vi "LH_DeleteIndexedContent.vi"(0 "InputList":refnum<class "ListHead.lvclass">, 1 "Index":i32) -> (2 "OutputList":refnum<class "ListHead.lvclass">, 3 "OutputContent":i32, 4 "IsEmpty?":bool)   [LabVIEW 2014, in "ListHead.lvclass"]
uses:
  ListHead.lvclass
  ListHead.lvclass/ListHead.ctl
  ListNode.lvclass
  ListNodeVirtual.lvclass
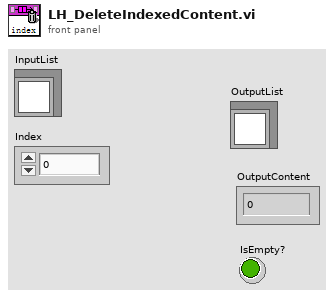
[diagram p1: front panel]
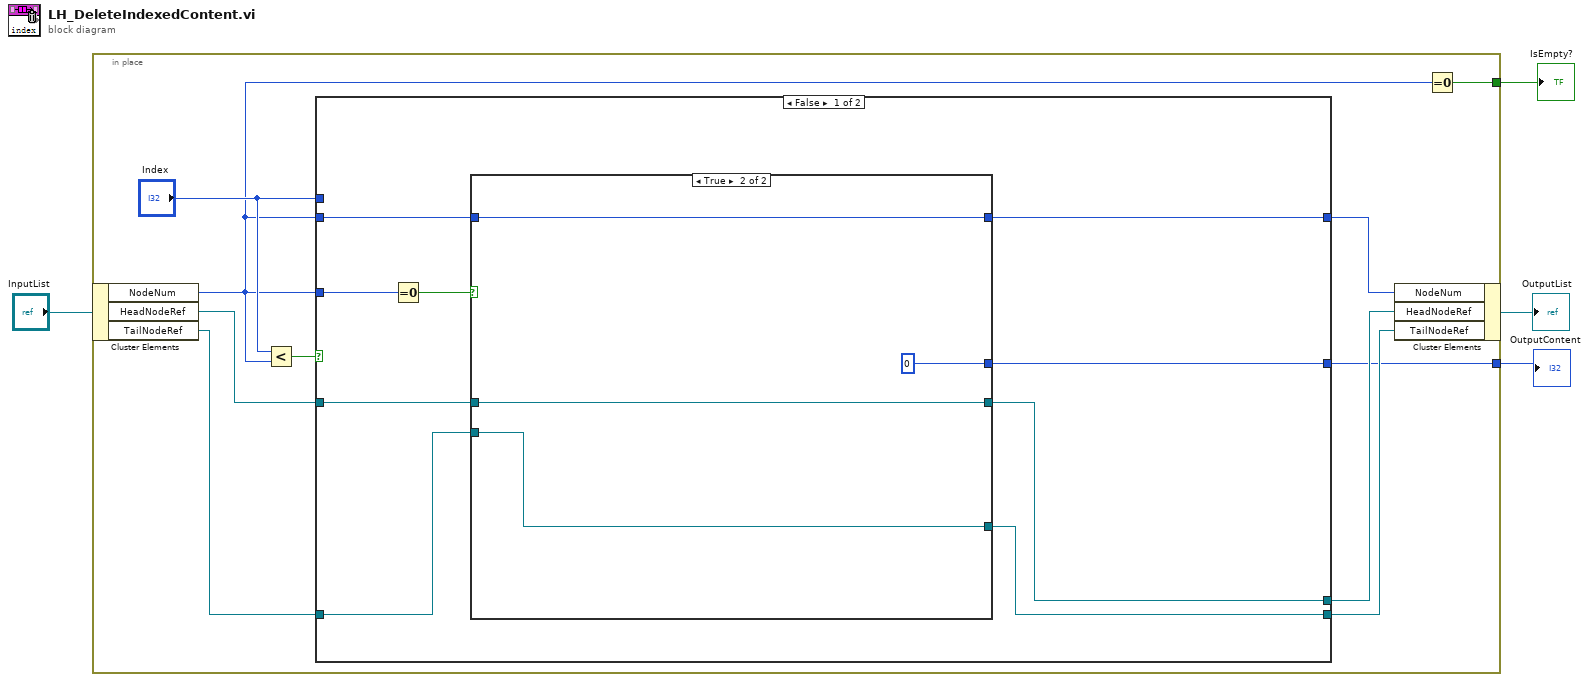
[diagram p0: block diagram]
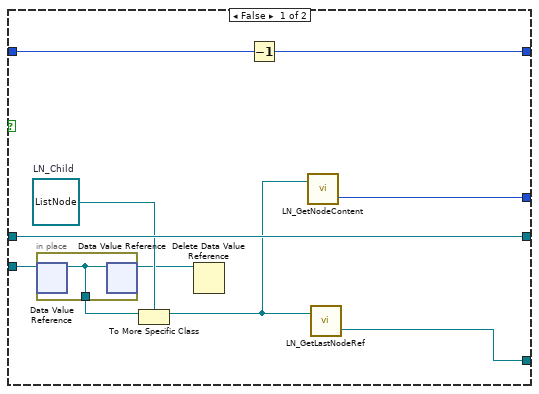
[diagram p2: hidden frame]
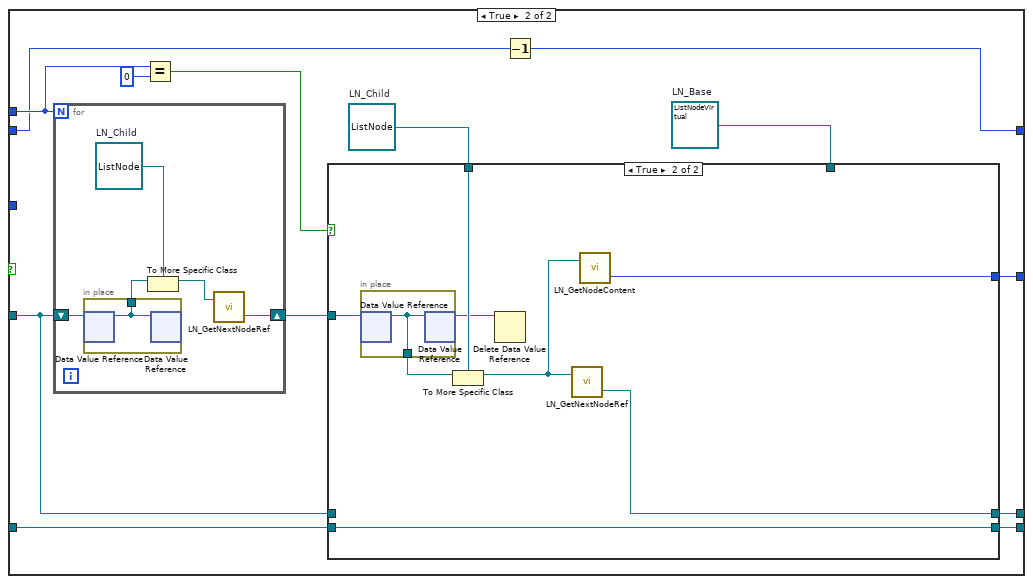
[diagram p3: hidden frame]
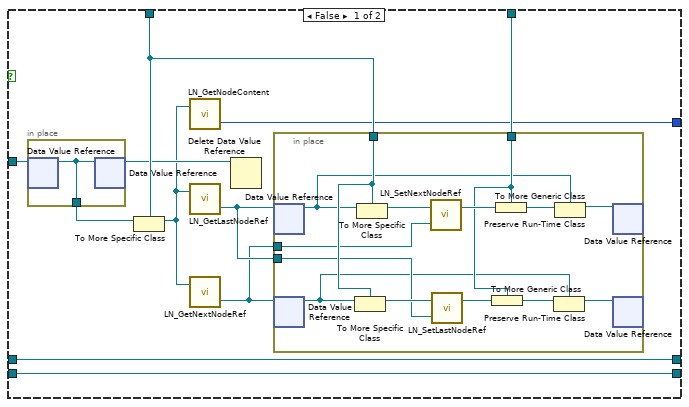
[diagram p4: hidden frame]
diagram:
  n1 = in-place {
    in-place-border: [w6] -> w2
    in-place-border: [w5] -> w1
    n2 = in-place-cluster #1("InputList") -> ("NodeNum"=w7:u32, "HeadNodeRef"=w13:refnum<data-value>, "TailNodeRef"=w12:refnum<data-value>)
    n3 = Less?(x="Index", y=w7) -> (x < y?=w14:bool)
    n4 = case shown="False" w14 {
      tunnel: w13 -> [w21 w43]
      tunnel: "Index" -> [_ w50]
      tunnel: w12 -> [w20 w41]
      tunnel: [w19 w42] -> w10
      tunnel: [w18 w40] -> w9
      tunnel: w7 -> [w23 _]
      tunnel: w7 -> [w17 w45]
      tunnel: [w16 w44] -> w8
      tunnel: [w15 w39] -> w5
      frame False {
        n5 = Equal To 0?(x=w23) -> (x = 0?=w22:bool)
        n6 = case shown="True" w22 {
          tunnel: w21 -> [w33 w38]
          tunnel: w20 -> [w32 w37]
          tunnel: [w28 w37] -> w18
          tunnel: [w33 w38] -> w19
          tunnel: w17 -> [w27 w36]
          tunnel: [w26 w36] -> w16
          tunnel: [w24 0 ("Content")] -> w15
          frame False {
            w31 = refnum<class "ListNode.lvclass"> refnum  # LN_Child
            n7 = in-place {
              in-place-border: [w34] -> w30
              n8 = in-place-dvr #2(w32) -> (w34:refnum<class "ListNodeVirtual.lvclass">)  [unwired: 1 out]
              n9 = in-place-dvr #2(w34) -> (w29:refnum<data-value>)  [unwired: 1 out]
            }
            n10 = To More Specific Class(target class=w31, reference=w30) -> (specific class reference=w25:refnum<class "ListNode.lvclass">)  [unwired: 1 in, 1 out]
            n11 = Delete Data Value Reference(data value reference=w29) -> ()  [unwired: 1 in, 2 out]
            n12 = Decrement(x=w27) -> (x-1=w26:u32)
            n13 = call "LN_GetNodeContent.vi"("InputNode"=w25) -> ("Content"=w24:i32)  [unwired: 1 in, 1 out]
            n14 = call "LN_GetLastNodeRef.vi"("InputListNode"=w25) -> ("OutputLastNodeRef"=w28:refnum<data-value>)  [unwired: 1 in, 1 out]
          }
          frame True {
          }
        }
      }
      frame True {
        w46 = refnum<class "ListNodeVirtual.lvclass"> refnum  # LN_Base
        w47 = refnum<class "ListNode.lvclass"> refnum  # LN_Child
        n15 = for {
          N: w50 -> [_]
          shift-right: [w87] -> w51
          shift-left: w43 -> [w91]
          w90 = refnum<class "ListNode.lvclass"> refnum  # LN_Child
          n16 = in-place {
            in-place-border: [w92] -> w89
            n17 = in-place-dvr #3(w91) -> (w92:refnum<class "ListNodeVirtual.lvclass">)  [unwired: 1 out]
            n18 = in-place-dvr #3(w92) -> ()  [unwired: 2 out]
          }
          n19 = To More Specific Class(target class=w90, reference=w89) -> (specific class reference=w88:refnum<class "ListNode.lvclass">)  [unwired: 1 in, 1 out]
          n20 = call "LN_GetNextNodeRef.vi"("InputListNode"=w88) -> ("OutputNextNodeRef"=w87:refnum<data-value>)  [unwired: 1 in, 1 out]
        }
        n21 = Equal?(x=w50, y=0) -> (x = y?=w48:bool)
        n22 = case shown="True" w48 {
          tunnel: w47 -> [w58 w84]
          tunnel: w51 -> [w61 w85]
          tunnel: w46 -> [w55 _]
          tunnel: w43 -> [w59 _]
          tunnel: [w59 w80] -> w42
          tunnel: w41 -> [w62 w81]
          tunnel: [w62 w81] -> w40
          tunnel: [w52 w78] -> w39
          frame False {
            n23 = in-place {
              in-place-border: [w77] -> w60
              n24 = in-place-dvr #4(w61) -> (w77:refnum<class "ListNodeVirtual.lvclass">)  [unwired: 1 out]
              n25 = in-place-dvr #4(w77) -> (w54:refnum<data-value>)  [unwired: 1 out]
            }
            n26 = To More Specific Class(target class=w58, reference=w60) -> (specific class reference=w53:refnum<class "ListNode.lvclass">)  [unwired: 1 in, 1 out]
            n27 = call "LN_GetNodeContent.vi"("InputNode"=w53) -> ("Content"=w52:i32)  [unwired: 1 in, 1 out]
            n28 = call "LN_GetLastNodeRef.vi"("InputListNode"=w53) -> ("OutputLastNodeRef"=w57:refnum<data-value>)  [unwired: 1 in, 1 out]
            n29 = call "LN_GetNextNodeRef.vi"("InputListNode"=w53) -> ("OutputNextNodeRef"=w56:refnum<data-value>)  [unwired: 1 in, 1 out]
            n30 = Delete Data Value Reference(data value reference=w54) -> ()  [unwired: 1 in, 2 out]
            n31 = in-place {
              in-place-border: w58 -> [w75]
              in-place-border: w57 -> [w72]
              in-place-border: w56 -> [w73]
              in-place-border: w55 -> [w69]
              n32 = in-place-dvr #5(w57) -> (w65:refnum<class "ListNodeVirtual.lvclass">)  [unwired: 1 out]
              n33 = in-place-dvr #6(w56) -> (w66:refnum<class "ListNodeVirtual.lvclass">)  [unwired: 1 out]
              n34 = To More Specific Class(target class=w75, reference=w66) -> (specific class reference=w76:refnum<class "ListNode.lvclass">)  [unwired: 1 in, 1 out]
              n35 = To More Specific Class(target class=w75, reference=w65) -> (specific class reference=w74:refnum<class "ListNode.lvclass">)  [unwired: 1 in, 1 out]
              n36 = call "LN_SetNextNodeRef.vi"("InputNextNodeRef"=w73, "InputListNode"=w74) -> ("OutputListNode"=w71:refnum<class "ListNode.lvclass">)  [unwired: 1 in]
              n37 = call "LN_SetLastNodeRef.vi"("InputLastNodeRef"=w72, "InputListNode"=w76) -> ("OutputListNode"=w70:refnum<class "ListNode.lvclass">)  [unwired: 1 in]
              n38 = To More Generic Class(target class=w69, reference=w70) -> (generic class reference=w67:refnum<class "ListNodeVirtual.lvclass">)
              n39 = To More Generic Class(target class=w69, reference=w71) -> (generic class reference=w68:refnum<class "ListNodeVirtual.lvclass">)
              n40 = Preserve Run-Time Class(object in=w67, 2:w66) -> (object out=w63:refnum<class "ListNodeVirtual.lvclass">)  [unwired: 1 in, 1 out]
              n41 = Preserve Run-Time Class(object in=w68, 2:w65) -> (object out=w64:refnum<class "ListNodeVirtual.lvclass">)  [unwired: 1 in, 1 out]
              n42 = in-place-dvr #5(w64) -> ()  [unwired: 2 out]
              n43 = in-place-dvr #6(w63) -> ()  [unwired: 2 out]
            }
          }
          frame True {
            n44 = in-place {
              in-place-border: [w86] -> w83
              n45 = in-place-dvr #7(w85) -> (w86:refnum<class "ListNodeVirtual.lvclass">)  [unwired: 1 out]
              n46 = in-place-dvr #7(w86) -> (w82:refnum<data-value>)  [unwired: 1 out]
            }
            n47 = To More Specific Class(target class=w84, reference=w83) -> (specific class reference=w79:refnum<class "ListNode.lvclass">)  [unwired: 1 in, 1 out]
            n48 = Delete Data Value Reference(data value reference=w82) -> ()  [unwired: 1 in, 2 out]
            n49 = call "LN_GetNextNodeRef.vi"("InputListNode"=w79) -> ("OutputNextNodeRef"=w80:refnum<data-value>)  [unwired: 1 in, 1 out]
            n50 = call "LN_GetNodeContent.vi"("InputNode"=w79) -> ("Content"=w78:i32)  [unwired: 1 in, 1 out]
          }
        }
        n51 = Decrement(x=w45) -> (x-1=w44:u32)
      }
    }
    n52 = in-place-cluster #1("NodeNum"=w8, "HeadNodeRef"=w10, "TailNodeRef"=w9) -> (→"OutputList":refnum<class "ListHead.lvclass">)
    n53 = Equal To 0?(x=w7) -> (x = 0?=w6:bool)
  }
  "IsEmpty?" <- w2
  "OutputContent" <- w1
